vi "Load all Device classes.vi"(8 "Error In":errorcluster) -> (0 "Error Out":errorcluster, 2 "Device Classes":refnum<class "Device.lvclass">[](array[class]), 3 "Device names":string[](array[string]))   [LabVIEW 2020, in "Test Framework.lvclass"]
uses:
  Test Framework.lvclass
  Devices/Device.lvclass
  Devices/Controls/Device Information Cluster.ctl
  Devices/Controls/Register to Write.ctl
  Devices/PIC-device/PIC-Device.lvclass
panel:
  out "Number of devices":i32
  out "All device names":string[](array[string])
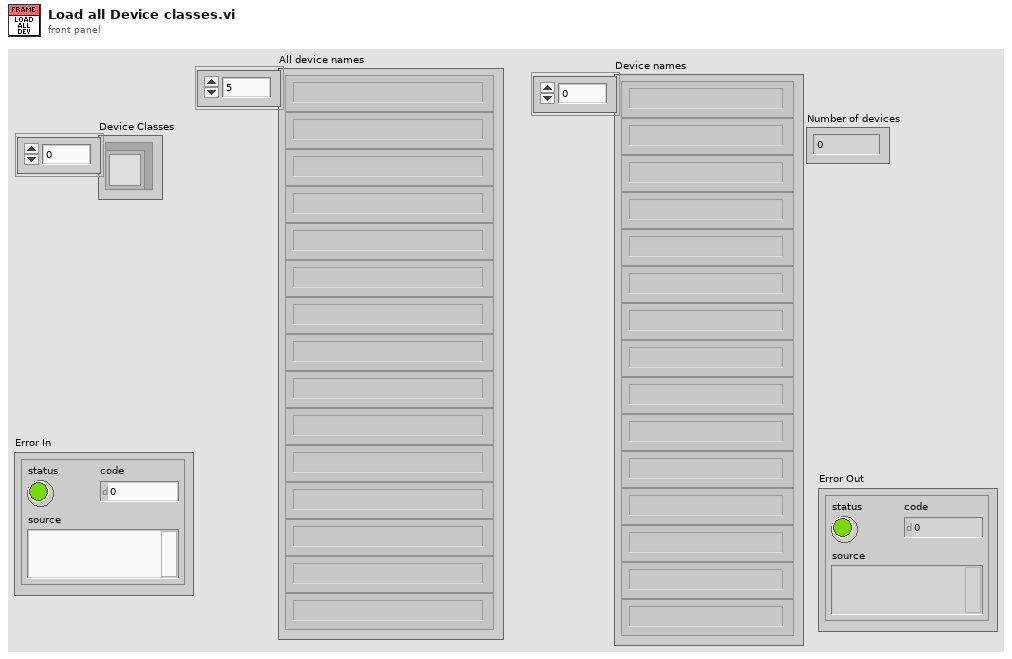
[diagram p1: front panel]
types:
  T1 = typedef "Device.lvclass/Device Information Cluster.ctl" = cluster{"Device Info":string[][], "Default Values":T2[], "Fetched info":string[][]}
  T2 = typedef "PIC-Device.lvclass/Register to Write.ctl" = cluster{"Register":u32, "Value":u32, "Dev Address":u32, "Physical Adress":u32}
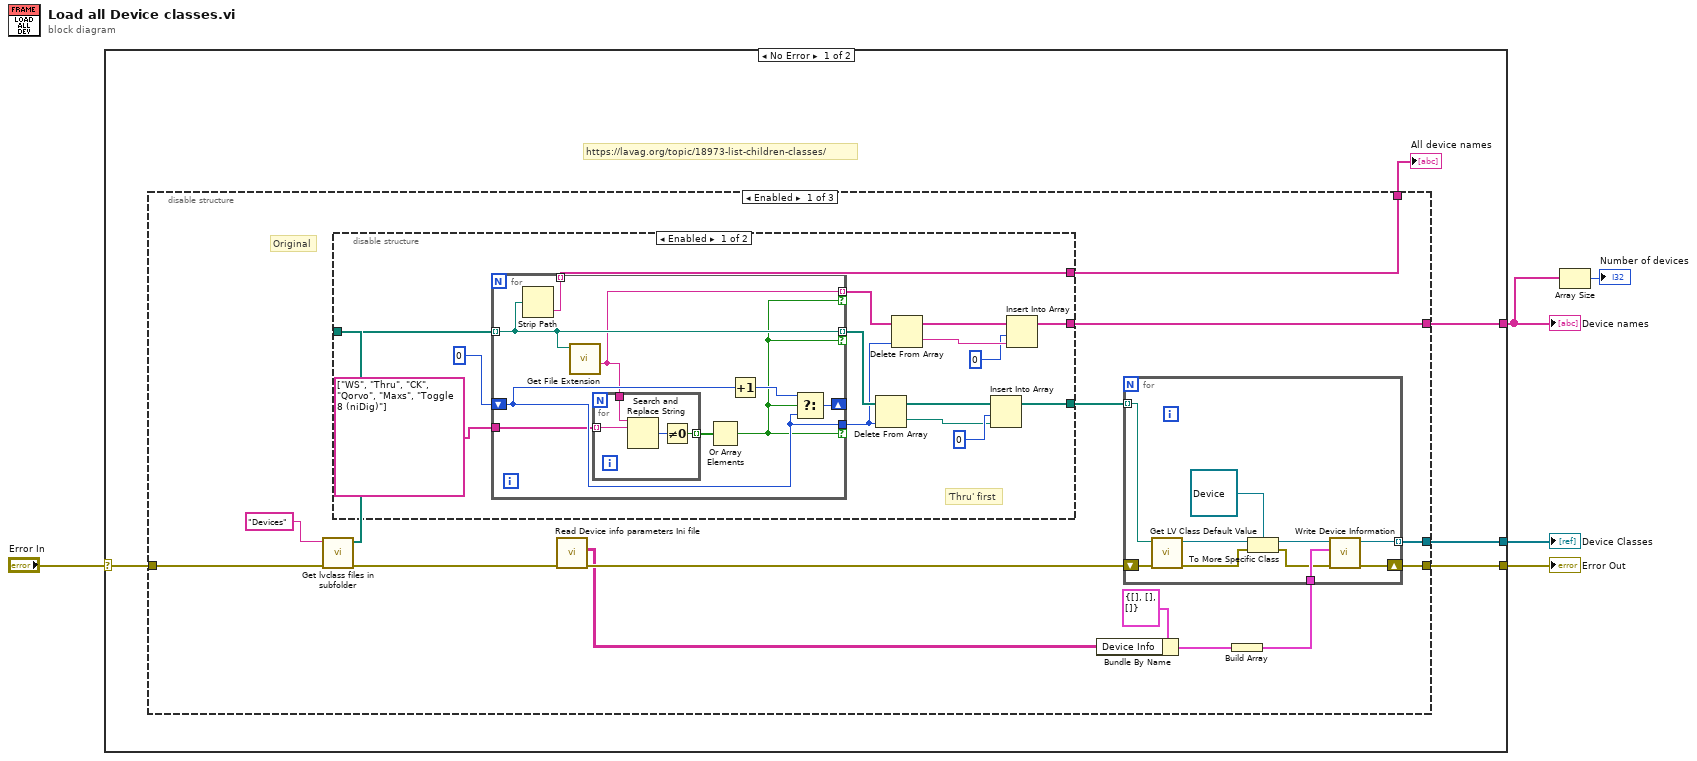
[diagram p0: block diagram]
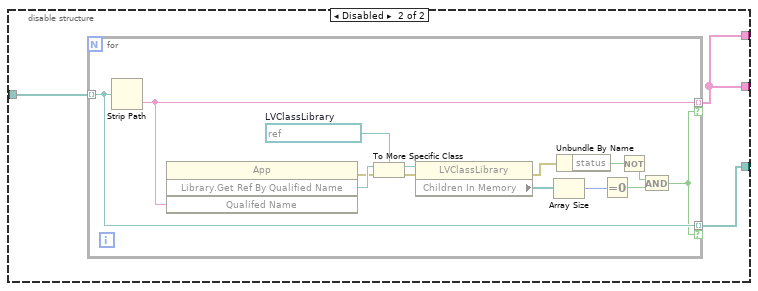
[diagram p2: hidden frame]
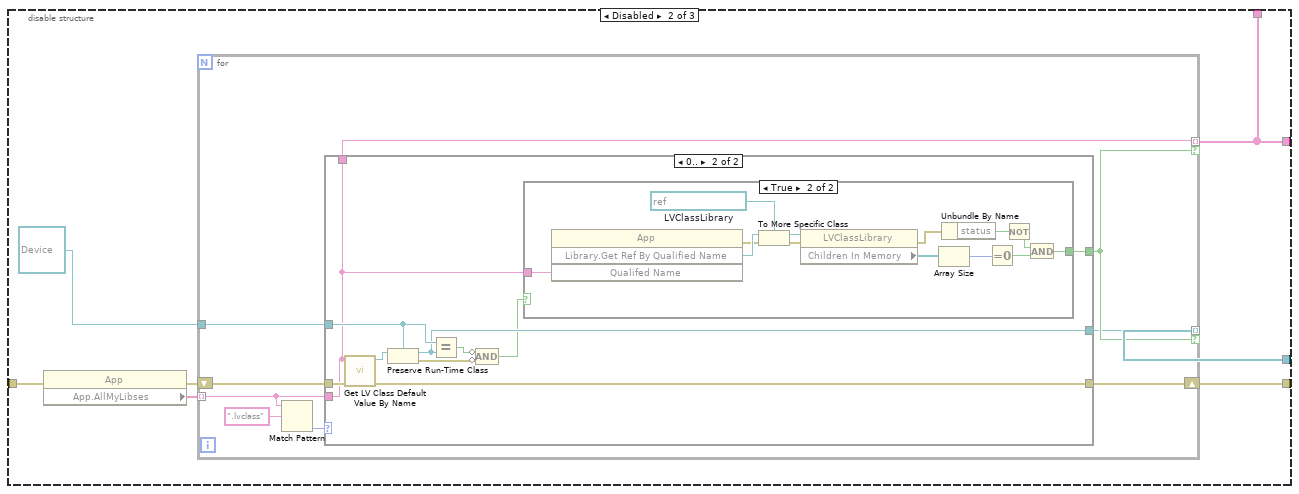
[diagram p3: hidden frame]
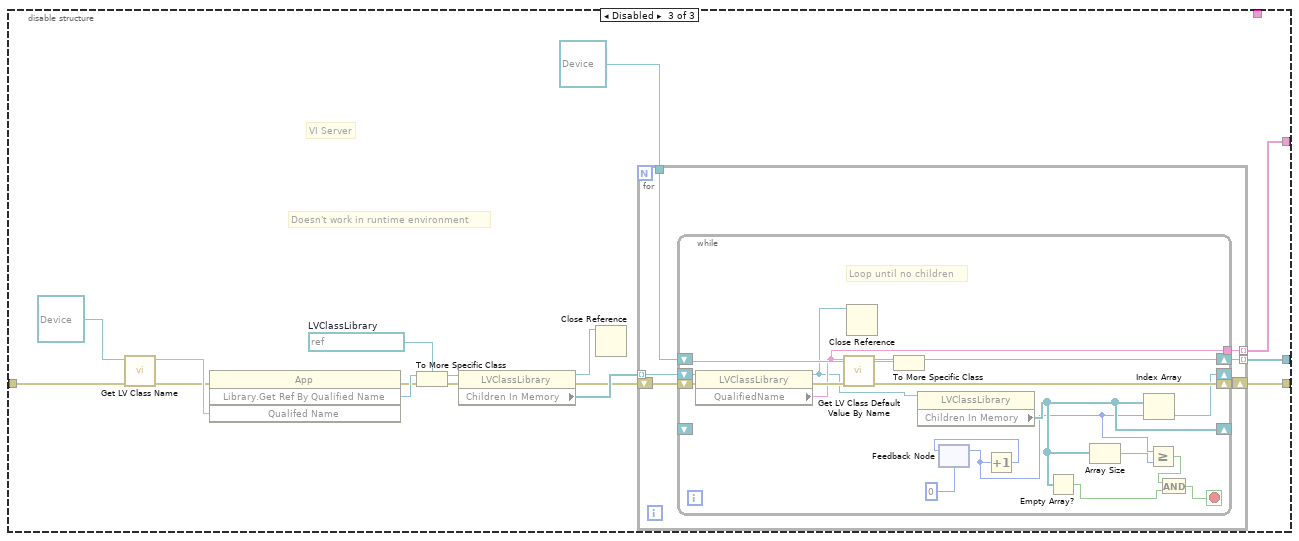
[diagram p6: hidden frame]
diagram:
  n1 = case shown="No Error" "Error In" {
    selector: "Error In" -> [w10 w162]
    tunnel: [w9 _] -> w3
    tunnel: [w8 w162] -> w4
    tunnel: [w7 _] -> w2
    frame No Error {
      # "https://lavag.org/topic/18973-list-children-classes/"
      n2 = disable-structure shown="Enabled" {
        disable-tunnel: w10 -> [w24 w83 w123]
        disable-tunnel: [w21 w81 w124] -> w9
        disable-tunnel: [w20 w82 w127] -> w8
        disable-tunnel: [w12 w80 w122] -> w7
        disable-tunnel: [w11 w80 _] -> w6
        frame Enabled {
          # "Original"
          n3 = call "Get lvclass files in subfolder.vi"("Error In"=w24, "Sub Folder"="Devices") -> ("Error Out"=w19:errorcluster, "Found lvclass files"=w22:path[])  [unwired: 8 in]
          n4 = disable-structure shown="Enabled" {
            disable-tunnel: w22 -> [w39 w54]
            disable-tunnel: [w38 w53] -> w13
            disable-tunnel: [w28 w55] -> w12
            disable-tunnel: [w26 w55] -> w11
            frame Enabled {
              # "'Thru' first"
              n5 = for {
                tunnel: w39 -> [w45] mode=indexing
                tunnel: [w45] -> w34 mode=indexing if=w40
                tunnel: [w43] -> w29 mode=indexing if=w40
                tunnel: [w46] -> w27 if=w40
                shift-right: [w48] -> _
                shift-left: 0 -> [w46]
                tunnel: [w44] -> w26 mode=indexing
                tunnel: string[] ["WS", "Thru", "CK", "Qorvo", "Maxs", "Toggle 8 (niDig)"] -> [w42]
                n6 = Strip Path(path=w45) -> (name=w44:string)  [unwired: 1 out]
                n7 = call <vilib>:"Get File Extension.vi"("file"=w45) -> ("filename without extension"=w43:string)  [unwired: 6 in, 4 out]
                n8 = for {
                  tunnel: [w51] -> w41 mode=indexing
                  tunnel: w43 -> [w50]
                  tunnel: w42 -> [w49] mode=indexing
                  n9 = Search and Replace String(input string=w50, search string=w49) -> (number of replacements=w52:i32)  [unwired: 6 in, 3 out]
                  n10 = Not Equal To 0?(x=w52) -> (x != 0?=w51:bool)
                }
                n11 = Or Array Elements(Boolean array=w41) -> (logical OR=w40:bool)
                n12 = Increment(x=w46) -> (x+1=w47:i32)
                n13 = Select(t=w47, s=w40, f=w46) -> (s? t:f=w48:i32)
              }
              n14 = Delete From Array(array=w34, index=w27) -> (deleted portion=w35:path, array with subset deleted=w33:path[])  [unwired: 1 in]
              n15 = Delete From Array(array=w29, index=w27) -> (deleted portion=w31:string, array with subset deleted=w32:string[])  [unwired: 1 in]
              n16 = Insert Into Array(array=w33, index=0, new element=w35) -> (w38:path[])
              n17 = Insert Into Array(array=w32, index=0, new element=w31) -> (w28:string[])
            }
            frame Disabled {
              n18 = for {
                tunnel: w54 -> [w57] mode=indexing
                tunnel: [w69] -> w55 mode=indexing if=w56
                tunnel: [w57] -> w53 mode=indexing if=w56
                w66 = refnum<vi> refnum  # LVClassLibrary
                n19 = Strip Path(path=w57) -> (name=w69:string)  [unwired: 1 out]
                n20 = invoke class="App" method="Library.Get Ref By Qualified Name"("Qualifed Name"=w69) -> (error out=w67:errorcluster, "Library.Get Ref By Qualified Name"=w68:refnum<vi>)  [unwired: 3 in, 2 out]
                n21 = To More Specific Class(target class=w66, reference=w68, error in=w67) -> (specific class reference=w65:refnum<vi>, error out=w64:errorcluster)
                n22 = property class="LVClassLibrary"(reference=w65, error in=w64) -> (error out=w61:errorcluster, "Children In Memory"=w63:refnum<vi>[])  [unwired: 1 out]
                n23 = Array Size(array=w63) -> (size(s)=w62:i32)
                n24 = Unbundle By Name(w61) -> ("status"=w60:bool)
                n25 = Equal To 0?(x=w62) -> (x = 0?=w58:bool)
                n26 = Not(x=w60) -> (.not. x?=w59:bool)
                n27 = And(x=w59, y=w58) -> (x .and. y?=w56:bool)
              }
            }
          }
          n28 = call "Read Device info parameters Ini file.vi"("Error In"=w19) -> ("Error Out"=w18:errorcluster, "Parameter names only"=w14:string[][])  [unwired: 7 in, 2 out]
          n29 = Bundle By Name(cluster=T1 {"Device Info"=[], "Default Values"=[], "Fetched info"=[]} ("Device Defaults"), "Device Info"=w14) -> (w16:T1)
          n30 = Build Array(w16) -> (w15:T1[])
          n31 = for {
            tunnel: w13 -> [w78] mode=indexing
            shift-right: [w72] -> w20
            shift-left: w18 -> [w79]
            tunnel: [w73] -> w21 mode=indexing
            tunnel: w15 -> [w76]
            n32 = call <vilib>:"Get LV Class Default Value.vi"("error in (no error)"=w79, "class path"=w78) -> ("error out"=w77:errorcluster, "object"=w71:refnum<class>)  [unwired: 8 in]
            n33 = To More Specific Class(target class=refnum<class "Device.lvclass"> refnum ("Device.lvclass"), reference=w71, error in=w77) -> (specific class reference=w75:refnum<class "Device.lvclass">, error out=w74:errorcluster)
            n34 = call-dynamic "Write Device Information.vi"("error in (no error)"=w74, "Device Info"=w76, "Device in"=w75) -> ("error out"=w72:errorcluster, "Device out"=w73:refnum<class "Device.lvclass">)  [unwired: 7 in]
          }
        }
        frame Disabled {
          n35 = property class="App"(error in=w83) -> (error out=w85:errorcluster, "App.AllMyLibses"=w86:string[])  [unwired: 1 in, 1 out]
          n36 = for {
            tunnel: w86 -> [w92] mode=indexing
            tunnel: refnum<class "Device.lvclass"> refnum ("Device.lvclass") -> [w93]
            shift-right: [w90] -> w82
            shift-left: w85 -> [w91]
            tunnel: [w88] -> w81 mode=indexing if=w89
            tunnel: [w87] -> w80 mode=indexing if=w89
            n37 = Match Pattern(string=w92, regular expression=".lvclass") -> (offset past match=w94:i32)  [unwired: 1 in, 3 out]
            n38 = case shown="0.." w94 {
              tunnel: w93 -> [_ w104]
              tunnel: w92 -> [w96 w100]
              tunnel: w91 -> [w97 w107]
              tunnel: [w97 w106] -> w90
              tunnel: [_ w103] -> w88
              tunnel: [_ w98] -> w89
              tunnel: [w96 w100] -> w87
              frame Default {
              }
              frame 0.. {
                n39 = call <vilib>:"Get LV Class Default Value By Name.vi"("error in (no error)"=w107, "class name"=w100) -> ("error out"=w106:errorcluster, "object"=w105:refnum<class>)  [unwired: 8 in]
                n40 = Preserve Run-Time Class(object in=w105, 2:w104) -> (object out=w103:refnum<class "Device.lvclass">, error out=w102:errorcluster)  [unwired: 1 in]
                n41 = Equal?(x=w104, y=w103) -> (x = y?=w101:bool)
                n42 = Compound Arithmetic op=AND(invert w101, invert w102) -> (w99:bool)
                n43 = case shown="True" w99 {
                  selector: w99 -> [w108 _]
                  tunnel: w100 -> [_ w115]
                  tunnel: [w108 w109] -> w98
                  frame False {
                  }
                  frame True {
                    w119 = refnum<vi> refnum  # LVClassLibrary
                    n44 = invoke class="App" method="Library.Get Ref By Qualified Name"("Qualifed Name"=w115) -> (error out=w120:errorcluster, "Library.Get Ref By Qualified Name"=w121:refnum<vi>)  [unwired: 3 in, 2 out]
                    n45 = To More Specific Class(target class=w119, reference=w121, error in=w120) -> (specific class reference=w118:refnum<vi>, error out=w117:errorcluster)
                    n46 = property class="LVClassLibrary"(reference=w118, error in=w117) -> (error out=w113:errorcluster, "Children In Memory"=w116:refnum<vi>[])  [unwired: 1 out]
                    n47 = Array Size(array=w116) -> (size(s)=w114:i32)
                    n48 = Unbundle By Name(w113) -> ("status"=w112:bool)
                    n49 = Equal To 0?(x=w114) -> (x = 0?=w110:bool)
                    n50 = Not(x=w112) -> (.not. x?=w111:bool)
                    n51 = And(x=w111, y=w110) -> (x .and. y?=w109:bool)
                  }
                }
              }
            }
          }
        }
        frame Disabled {
          w132 = refnum<vi> refnum  # LVClassLibrary
          # "Doesn't work in runtime environment"
          # "VI Server"
          n52 = call <vilib>:"Get LV Class Name.vi"("error in (no error)"=w123, "object"=refnum<class "Device.lvclass"> refnum ("Device.lvclass")) -> ("error out"=w133:errorcluster, "class name"=w136:string)  [unwired: 8 in]
          n53 = invoke class="App" method="Library.Get Ref By Qualified Name"(error in=w133, "Qualifed Name"=w136) -> (error out=w134:errorcluster, "Library.Get Ref By Qualified Name"=w135:refnum<vi>)  [unwired: 2 in, 2 out]
          n54 = To More Specific Class(target class=w132, reference=w135, error in=w134) -> (specific class reference=w131:refnum<vi>, error out=w130:errorcluster)
          n55 = property class="LVClassLibrary"(reference=w131, error in=w130) -> (reference out=w129:refnum<vi>, error out=w126:errorcluster, "Children In Memory"=w128:refnum<vi>[])
          n56 = Close Reference(reference=w129) -> ()  [unwired: 1 in, 1 out]
          n57 = for {
            tunnel: w128 -> [w143] mode=indexing
            tunnel: refnum<class "Device.lvclass"> refnum ("Device.lvclass") -> [w140]
            tunnel: [w139] -> w124 mode=indexing
            shift-right: [w142] -> w127
            shift-left: w126 -> [w141]
            tunnel: [w138] -> w122 mode=indexing
            n58 = while {
              tunnel: [w154] -> w138
              shift-right: [w160] -> w142
              shift-left: w141 -> [w158]
              shift-right: [w155] -> w139
              shift-left: w140 -> [w157]
              shift-right: [w152] -> _
              shift-left: w143 -> [w161]
              shift-right: [w149] -> _
              shift-left: _ -> [_]
              stop <- w144 stop-if-true
              # "Loop until no children"
              n59 = property class="LVClassLibrary"(reference=w161, error in=w158) -> (reference out=w153:refnum<vi>, error out=w159:errorcluster, "QualifiedName"=w154:string)
              n60 = call <vilib>:"Get LV Class Default Value By Name.vi"("error in (no error)"=w159, "class name"=w154) -> ("error out"=w160:errorcluster, "object"=w156:refnum<class>)  [unwired: 8 in]
              n61 = Close Reference(reference=w153) -> ()  [unwired: 1 in, 1 out]
              n62 = To More Specific Class(target class=w157, reference=w156) -> (specific class reference=w155:refnum<class "Device.lvclass">)  [unwired: 1 in, 1 out]
              n63 = property class="LVClassLibrary"(reference=w153) -> ("Children In Memory"=w149:refnum<vi>[])  [unwired: 1 in, 2 out]
              n64 = feedback #1(0) -> (w147:i32)
              n65 = Increment(x=w147) -> (x+1=w150:i32)
              n66 = feedback-in #1(w150) -> ()
              n67 = Empty Array?(array=w149) -> (empty?=w146:bool)
              n68 = Array Size(array=w149) -> (size(s)=w148:i32)
              n69 = Index Array(array=w149, index=w147) -> (element=w152:refnum<vi>)
              n70 = Greater Or Equal?(x=w147, y=w148) -> (x >= y?=w145:bool)
              n71 = And(x=w145, y=w146) -> (x .and. y?=w144:bool)
            }
          }
        }
      }
      "All device names" <- w6
    }
    frame Error {
    }
  }
  "Error Out" <- w4
  "Device names" <- w2
  "Device Classes" <- w3
  n72 = Array Size(array=w2) -> (size(s)=→"Number of devices":i32)
